vi "Pause_for_server_ch_val.vi"(2 "Extra command string":string, 3 "Simulate/Run":T1) -> (0 "Extra command string Out":string, 1 "Error Comments":string)   [LabVIEW 2022 SP3]
uses:
  Controls/User_Specific_mode.ctl
  ADAM Client/Sub VIs/ADAM Controls/Channel_names.ctl
  Globals/Extra_Commands_Global.vi
panel:
  out "Operator":string
  out "Minutes Waited":dbl format="%.2f"
  out "Channel Found?":bool
  out "Time to email next":dbl format="%.2f"
  out "Actual Value":string
  out "Channel Value":string
  out "Channel Name":string
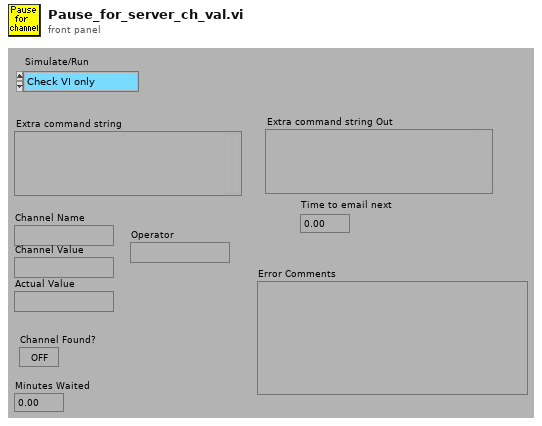
[diagram p1: front panel]
types:
  T1 = typedef "User_Specific_mode.ctl" = enum16{"Check VI only", "Run VI"}
  T2 = typedef "Channel_names.ctl" = enum16{"Active Only", "Active + Off", "All Channels", "Changeable Only"}
  T3 = typedef "Ch_description_ADAM.ctl" = cluster{"Ch Name":string, "Type":T4, "Function":T5, "Ch State":T6, "Calibration type":T7, "A":dbl, "B":dbl, "C":dbl, "D":dbl, "Comments":string, "Address":T8, "String":string, "Duty":u16}
  T4 = typedef "Module_type_ADAM.ctl" = string
  T5 = typedef "Function_ADAM.ctl" = enum16{"Analogue Input", "Digital Input", "Event counter", "Event rate", "Analogue Output", "Digital Output", "Relay Output"}
  T6 = typedef "Channel_State.ctl" = enum16{"On", "Off", "Always On", "Always Off"}
  T7 = typedef "Calib_type_ADAM.ctl" = string
  T8 = typedef "Address.ctl" = cluster{"Main":i32, "Ch.":i32, "Sub":i32, "Port Name":string}
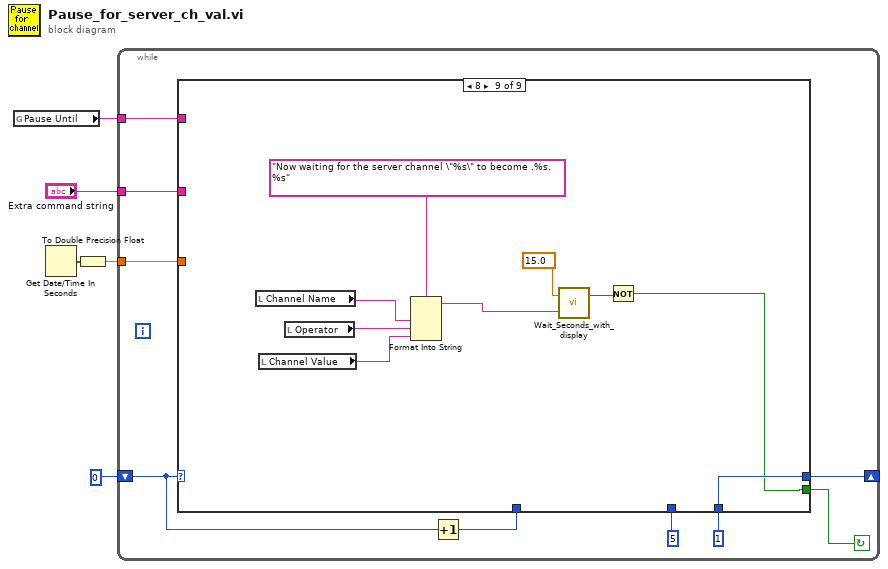
[diagram p0: block diagram]
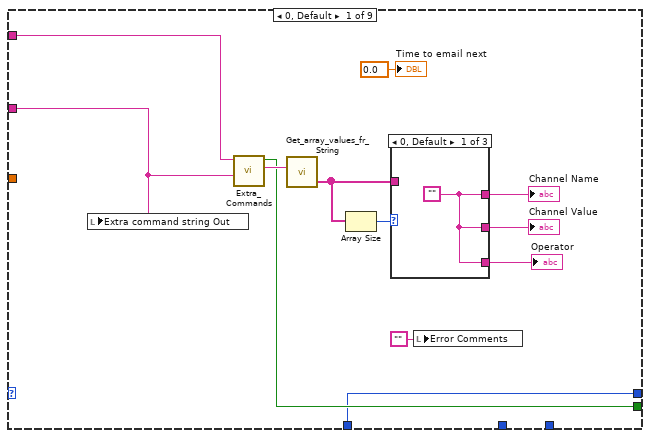
[diagram p2: hidden frame]
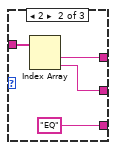
[diagram p3: hidden frame]
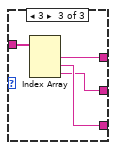
[diagram p4: hidden frame]
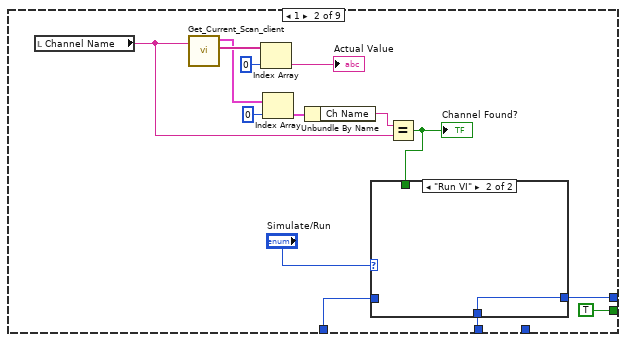
[diagram p5: hidden frame]
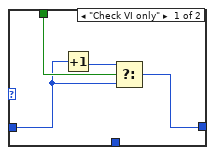
[diagram p6: hidden frame]
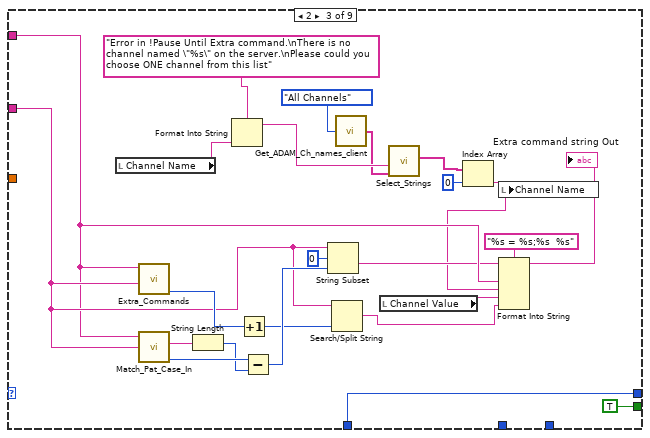
[diagram p7: hidden frame]
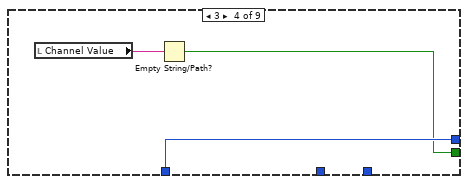
[diagram p8: hidden frame]
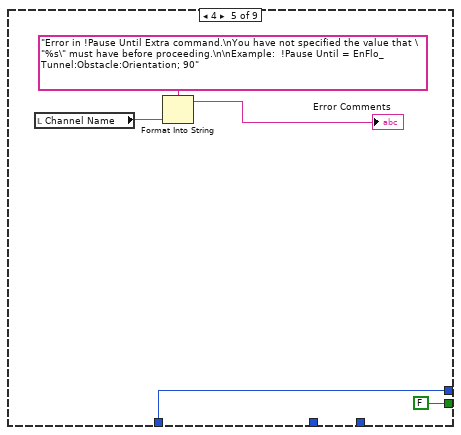
[diagram p9: hidden frame]
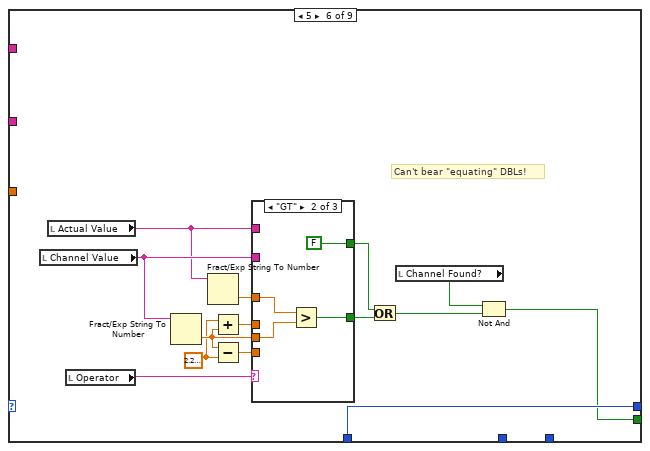
[diagram p10: hidden frame]
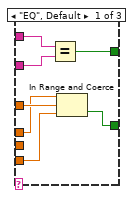
[diagram p11: hidden frame]
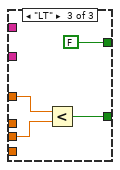
[diagram p12: hidden frame]
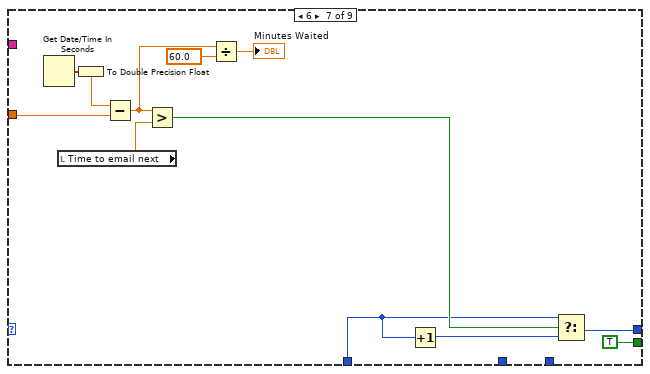
[diagram p13: hidden frame]
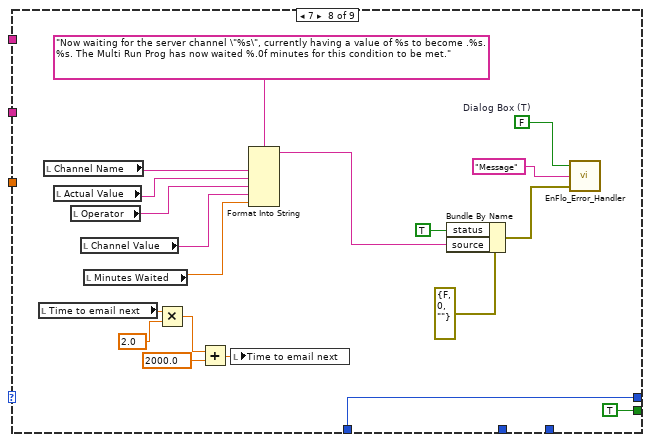
[diagram p14: hidden frame]
diagram:
  n1 = global read "Extra_Commands_Global.vi" "Pause Until"() -> (w3:string)
  n2 = Get Date/Time In Seconds() -> (seconds since 1Jan1904=w1:timestamp)
  n3 = To Double Precision Float(number=w1) -> (double precision float=w2:dbl)
  n4 = while {
    tunnel: w2 -> [w7]
    tunnel: w3 -> [w8]
    tunnel: "Extra command string" -> [w9]
    shift-left: 0 -> [w13]
    shift-right: [w11] -> _
    stop <- w14 continue-if-true
    n5 = Increment(x=w13) -> (x+1=w12:i32)
    n6 = case shown="8" w13 {
      tunnel: [w24 TRUE ("Command Found") TRUE ("Command Found") w79 FALSE ("Command Found") w98 TRUE ("Command Found") TRUE ("Command Found") w148] -> w14
      tunnel: w12 -> [w23 w40 w58 w81 w86 w100 w122 w146 _]
      tunnel: [w23 w39 w58 w81 w86 w100 w120 w146 w150] -> w11
      tunnel: 5 ("f") -> [_ w38 _ _ _ _ _ _ _]
      tunnel: w9 -> [w20 _ w65 _ _ _ _ _ _]
      tunnel: w8 -> [w21 _ w64 _ _ _ _ _ _]
      tunnel: w7 -> [_ _ _ _ _ _ w124 _ _]
      tunnel: 1 ("f") -> [_ _ _ _ _ _ _ _ w150]
      frame 0, Default {
        n7 = local write "Extra command string Out"(w20) -> ()
        n8 = call "Extra_Commands.vi"("String to Search"=w20, "Command"=w21) -> ("String Value"=w26:string, "Command Found"=w24:bool)  [unwired: 1 in, 3 out]
        n9 = call "Get_array_values_fr_String.vi"("String Value"=w26) -> ("String array"=w16:string[])  [unwired: 1 out]
        n10 = Array Size(array=w16) -> (size(s)=w17:i32)
        n11 = case shown="0, Default" w17 {
          tunnel: w16 -> [_ w31 w35]
          tunnel: [w27 w30 w34] -> w25
          tunnel: [w27 w29 w32] -> w18
          tunnel: [w27 "EQ" ("Operator") w33] -> w15
          frame 0, Default {
            w27 = ""
          }
          frame 2 {
            n12 = Index Array(array=w31) -> (element #1=w30:string, element #2=w29:string)  [unwired: 2 in]
          }
          frame 3 {
            n13 = Index Array(array=w35) -> (element #1=w34:string, element #2=w33:string, element #3=w32:string)  [unwired: 3 in]
          }
        }
        "Channel Name" <- w25
        "Channel Value" <- w18
        "Operator" <- w15
        n14 = local write "Error Comments"("") -> ()
        "Time to email next" <- 0.0 ("Time to email next")
      }
      frame 1 {
        n15 = local read "Channel Name"() -> (w36:string)
        n16 = call "Get_Current_Scan_client.vi"("singleChannel"=w36) -> ("Ch Description Array"=w46:T3[], "String values"=w49:string[])  [unwired: 1 in, 2 out]
        n17 = Index Array(array=w49, index=0 ("Index")) -> (element=→"Actual Value":string)
        n18 = Index Array(array=w46, index=0 ("Index")) -> (element=w45:T3)
        n19 = Unbundle By Name(w45) -> ("Ch Name"=w44:string)
        n20 = Equal?(x=w44, y=w36) -> (x = y?=w37:bool)
        "Channel Found?" <- w37
        n21 = case shown="\"Run VI\"" "Simulate/Run" {
          tunnel: w40 -> [w51 _]
          tunnel: [w50 w54] -> w39
          tunnel: w38 -> [_ w54]
          tunnel: w37 -> [w53 _]
          frame "Check VI only" {
            n22 = Increment(x=w51) -> (x+1=w52:i32)
            n23 = Select(t=w52, s=w53, f=w51) -> (s? t:f=w50:i32)
          }
          frame "Run VI" {
          }
        }
      }
      frame 2 {
        n24 = local read "Channel Name"() -> (w76:string)
        n25 = call "Extra_Commands.vi"("String to Search"=w65, "Command"=w64) -> ("Offset Past Command"=w66:i32)  [unwired: 1 in, 4 out]
        n26 = call "Match_Pat_Case_In.vi"("String to match"=w64, "String"=w65) -> ("Matched string"=w71:string, "offset past match"=w70:i32)  [unwired: 1 in, 2 out]
        n27 = String Length(string=w71) -> (length=w69:i32)
        n28 = Format Into String(format string="Error in !Pause Until Extra command.\nThere is no channel named \"%s\" on the server.\nPlease could you choose ONE channel from this list" ("Format String"), w76) -> (resulting string=w75:string)  [unwired: 2 in, 1 out]
        n29 = Increment(x=w66) -> (x+1=w56:i32)
        n30 = Subtract(x=w70, y=w69) -> (x-y=w68:i32)
        n31 = String Subset(string=w65, offset (0)=0, length (rest)=w68) -> (substring=w63:string)
        n32 = Search/Split String(string=w65, offset (0)=w56) -> (match + rest of string=w62:string)  [unwired: 3 out]
        n33 = call "Get_ADAM_Ch_names_client.vi"("Channel names set"=Channel_names."All Channels") -> ("Ch names"=w73:string[])
        n34 = local read "Channel Value"() -> (w59:string)
        n35 = call "Select_Strings.vi"("Available Ch names"=w73, "Message"=w75) -> ("Selected Channel Names"=w55:string[])  [unwired: 3 in, 3 out]
        n36 = Index Array(array=w55, index=0 ("Index")) -> (element=w57:string)
        n37 = local write "Channel Name"(w57) -> ()
        n38 = Format Into String(format string="%s = %s;%s  %s" ("Format String"), initial string=w63, w64, w57, w59, w62) -> (resulting string=→"Extra command string Out":string)  [unwired: 1 in, 1 out]
      }
      frame 3 {
        n39 = local read "Channel Value"() -> (w80:string)
        n40 = Empty String/Path?(string/path=w80) -> (empty?=w79:bool)
      }
      frame 4 {
        n41 = local read "Channel Name"() -> (w82:string)
        n42 = Format Into String(format string="Error in !Pause Until Extra command.\nYou have not specified the value that \"%s\" must have before proceeding.\n\nExample:  !Pause Until = EnFlo_Tunnel:Obstacle:Orientation; 90", w82) -> (resulting string=→"Error Comments":string)  [unwired: 2 in, 1 out]
      }
      frame 5 {
        w89 = 2.220446049250313e-16
        # "Can't bear \"equating\" DBLs!"
        n43 = local read "Channel Value"() -> (w93:string)
        n44 = local read "Actual Value"() -> (w92:string)
        n45 = local read "Operator"() -> (w94:string)
        n46 = Fract/Exp String To Number(string=w93) -> (number=w90:dbl)  [unwired: 4 out]
        n47 = Fract/Exp String To Number(string=w92) -> (number=w97:dbl)  [unwired: 4 out]
        n48 = Add(x=w89, y=w90) -> (x+y=w88:dbl)
        n49 = Subtract(x=w90, y=w89) -> (x-y=w87:dbl)
        n50 = case shown="\"GT\"" w94 {
          tunnel: w97 -> [w104 w111 w115]
          tunnel: w90 -> [_ w110 w114]
          tunnel: [w103 w109 w113] -> w96
          tunnel: w93 -> [w107 _ _]
          tunnel: w92 -> [w106 _ _]
          tunnel: [w105 FALSE FALSE] -> w91
          tunnel: w88 -> [w102 _ _]
          tunnel: w87 -> [w101 _ _]
          frame "EQ", Default {
            n51 = Equal?(x=w106, y=w107) -> (x = y?=w105:bool)
            n52 = In Range and Coerce(upper limit=w102, x=w104, lower limit=w101) -> (In Range?=w103:bool)  [unwired: 1 out]
          }
          frame "GT" {
            n53 = Greater?(x=w111, y=w110) -> (0:w109:bool)
          }
          frame "LT" {
            n54 = Less?(x=w115, y=w114) -> (x < y?=w113:bool)
          }
        }
        n55 = Or(x=w91, y=w96) -> (x .or. y?=w95:bool)
        n56 = local read "Channel Found?"() -> (w99:bool)
        n57 = Not And(1:w95, 2:w99) -> (0:w98:bool)
      }
      frame 6 {
        n58 = Get Date/Time In Seconds() -> (seconds since 1Jan1904=w116:timestamp)
        n59 = local read "Time to email next"() -> (w125:dbl)
        n60 = To Double Precision Float(number=w116) -> (double precision float=w126:dbl)
        n61 = Subtract(x=w126, y=w124) -> (x-y=w119:dbl)
        n62 = Greater?(x=w119, y=w125) -> (0:w123:bool)
        n63 = Divide(x=w119, y=60.0) -> (x/y=→"Minutes Waited":dbl)
        n64 = Increment(x=w122) -> (x+1=w121:i32)
        n65 = Select(t=w122, s=w123, f=w121) -> (s? t:f=w120:i32)
      }
      frame 7 {
        w142 = FALSE  # Dialog Box (T)
        n66 = local read "Time to email next"() -> (w135:dbl)
        n67 = local read "Channel Name"() -> (w130:string)
        n68 = local read "Actual Value"() -> (w141:string)
        n69 = local read "Operator"() -> (w129:string)
        n70 = local read "Channel Value"() -> (w128:string)
        n71 = local read "Minutes Waited"() -> (w140:dbl)
        n72 = Multiply(x=w135, y=2.0) -> (x*y=w133:dbl)
        n73 = Add(x=w133, y=2000.0) -> (x+y=w131:dbl)
        n74 = local write "Time to email next"(w131) -> ()
        n75 = Format Into String(format string="Now waiting for the server channel \"%s\", currently having a value of %s to become .%s. %s. The Multi Run Prog has now waited %.0f minutes for this condition to be met." ("Format String"), w130, w141, w129, w128, w140) -> (resulting string=w136:string)  [unwired: 2 in, 1 out]
        n76 = Bundle By Name(cluster=errorcluster {"status"=FALSE, "code"=0, "source"=""} ("error in (no error)"), "status"=TRUE ("Bundle Element"), "source"=w136) -> (w143:errorcluster)
        n77 = call "EnFlo_Error_Handler.vi"("error in (no error)"=w143, "Error Type"="Message", "Dialog Box (F)"=w142) -> ()  [unwired: 3 out]
      }
      frame 8 {
        n78 = local read "Channel Name"() -> (w154:string)
        n79 = local read "Channel Value"() -> (w153:string)
        n80 = local read "Operator"() -> (w147:string)
        n81 = Format Into String(format string="Now waiting for the server channel \"%s\" to become .%s. %s" ("Format String"), w154, w147, w153) -> (resulting string=w151:string)  [unwired: 2 in, 1 out]
        n82 = call "Wait_Seconds_with_display.vi"("Message"=w151, "Seconds to wait"=15.0) -> ("Stopped"=w149:bool)  [unwired: 1 out]
        n83 = Not(x=w149) -> (.not. x?=w148:bool)
      }
    }
  }
